vi "Analysis Results.vi"(6 "Image Nr":i32, 8 "error in (no error)":errorcluster, 9 "Results In":refnum<class "Analyze Results Base.lvclass">[](array[class]), 10 "Parameters":refnum<class "Analyze Parameter Base.lvclass">[](array[class]), 11 "HIJ Vision Display in":refnum<class "HIJ Vision Display.lvclass">) -> (0 "error out":errorcluster, 3 "HIJ Vision Display out":refnum<class "HIJ Vision Display.lvclass">)   [LabVIEW 2020, in "HIJ Vision Display.lvlib" / "HIJ Vision Display.lvclass"]
uses:
  HIJ Vision Display.lvclass
  HIJ Vision Display.lvclass/HIJ Vision Display.ctl
  Analyze/Results and Overlays/Results Base/Analyze Results Base.lvclass
  Analyze/Results and Overlays/Static Overlay/Static Overlay.lvclass
  Analyze/Analyze Parameter/Analyze Parameter Base/Analyze Parameter Base.lvclass
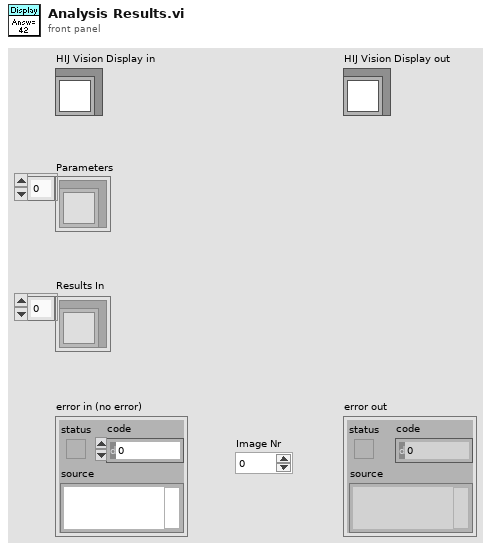
[diagram p1: front panel]
types:
  T1 = typedef "IMAQ Image.ctl" = refnum<image>
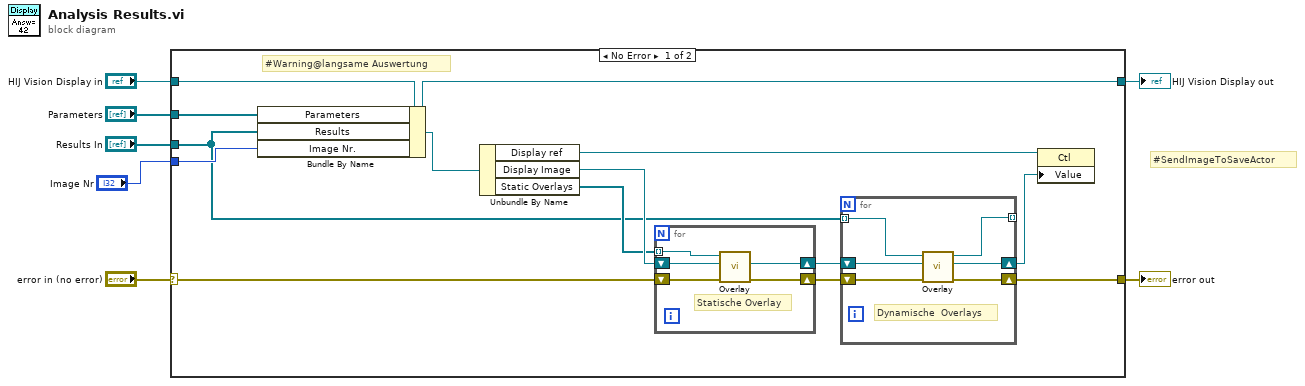
[diagram p0: block diagram]
diagram:
  # "#SendImageToSaveActor"
  n1 = case shown="No Error" "error in (no error)" {
    selector: "error in (no error)" -> [w10 w33]
    tunnel: [w14 w33] -> w6
    tunnel: [w18 w32] -> w4
    tunnel: "HIJ Vision Display in" -> [w20 w32]
    tunnel: "Results In" -> [w8 _]
    tunnel: "Image Nr" -> [w13 _]
    tunnel: "Parameters" -> [w17 _]
    frame No Error {
      # "#Warning@langsame Auswertung"
      n2 = Bundle By Name(cluster=w20, "Parameters"=w17, "Results"=w8, "Image Nr."=w13) -> (w18:refnum<class "HIJ Vision Display.lvclass">)
      n3 = Unbundle By Name(w18) -> ("Display ref"=w16:refnum<vi>, "Display Image"=w19:T1, "Static Overlays"=w12:refnum<class "Static Overlay.lvclass">[])
      n4 = for {
        tunnel: w12 -> [w25] mode=indexing
        shift-right: [w23] -> w11
        shift-left: w19 -> [w24]
        shift-right: [w21] -> w9
        shift-left: w10 -> [w22]
        # "Statische Overlay"
        n5 = call-dynamic "Overlay.vi"("error in (no error)"=w22, "Image In"=w24, "Overlay Base in"=w25) -> ("error out"=w21:errorcluster, "Image out"=w23:T1)  [unwired: 6 in, 1 out]
      }
      n6 = for {
        shift-right: [w30] -> w15
        shift-left: w11 -> [w27]
        tunnel: w8 -> [w31] mode=indexing
        tunnel: [w29] -> _ mode=indexing
        shift-right: [w28] -> w14
        shift-left: w9 -> [w26]
        # "Dynamische  Overlays"
        n7 = call-dynamic "Overlay.vi"("error in (no error)"=w26, "Image In"=w27, "Overlay Base in"=w31) -> ("error out"=w28:errorcluster, "Image out"=w30:T1, "Overlay Base out"=w29:refnum<class "Analyze Results Base.lvclass">)  [unwired: 6 in]
      }
      n8 = property class="Ctl"(reference=w16, "Value"=w15) -> ()  [unwired: 1 in, 2 out]
    }
    frame Error {
    }
  }
  "error out" <- w6
  "HIJ Vision Display out" <- w4
